vi "SubVI_1.vi"(9 "Step width":dbl=0.2, 10 "App":dbl=0.1, 11 "Points":i32=10) -> (3 "Disorder Pattern 2":dbl[](array[numeric]))   [LabVIEW 2019]
panel:
  in  "Set":bool
  in  "Generate":bool
  out "Disorder Pattern":dbl[](graph)=[1.0078411649904462, 1.0078411649904462, 0.9846991573254764, 0.9846991573254764, 0.9978814600222632, 0.9978814600222632, 0.9723089162683902, 0.9723089162683902, 1.011631648566163, 1.011631648566163]
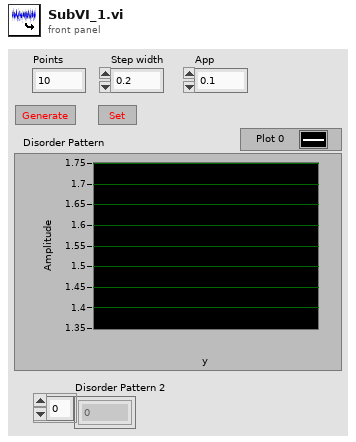
[diagram p1: front panel]
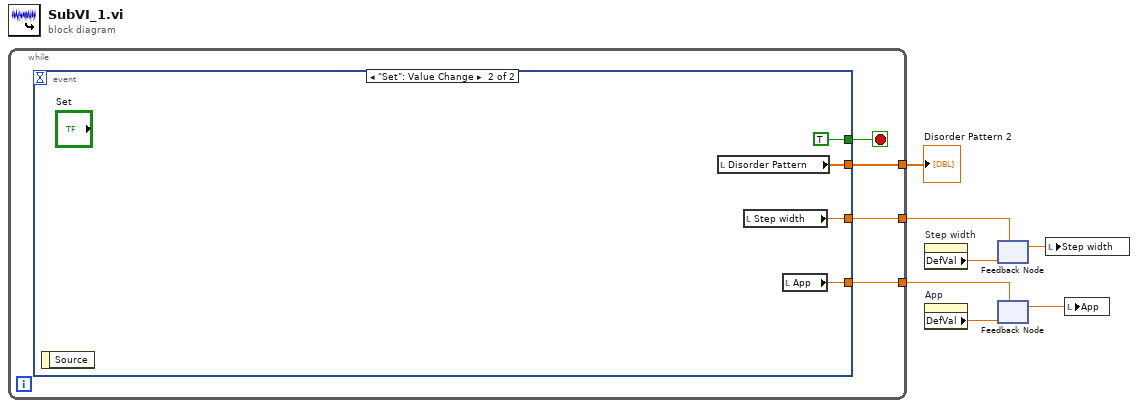
[diagram p0: block diagram]
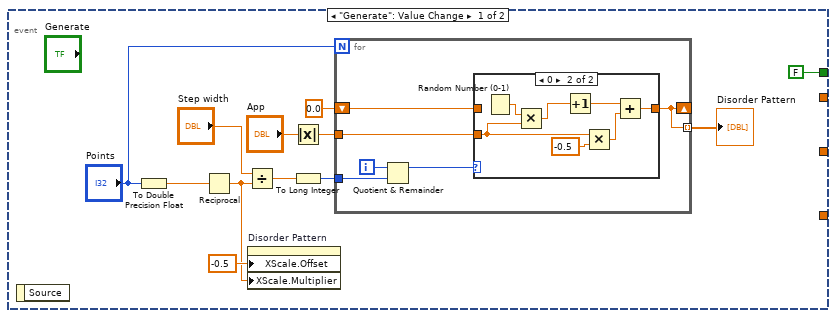
[diagram p2: hidden frame]
diagram:
  n1 = while {
    tunnel: [w10] -> w7
    tunnel: [w9] -> w4
    tunnel: [w8] -> w1
    stop <- w11 stop-if-true
    n2 = event shown="[1] \"Set\": Value Change" {
      selector: _ -> [_ _]
      dyn-events: _ -> [_ _]
      timeout: _ -> [_ _]
      tunnel: [FALSE TRUE] -> w11
      tunnel: [_ w41] -> w10
      tunnel: [_ w39] -> w9
      tunnel: [_ w38] -> w8
      event "Generate": Value Change {
        n3 = event-data() -> ()  [unwired: 1 in, 1 out]
        n4 = To Double Precision Float(number="Points") -> (double precision float=w17:dbl)
        n5 = Reciprocal(x=w17) -> (1/x=w12:dbl)
        n6 = Divide(x="Step width", y=w12) -> (x/y=w19:dbl)
        n7 = property on="Disorder Pattern" class="WFGraph (strict)"("XScale.Offset"=-0.5, "XScale.Multiplier"=w12) -> ()  [unwired: 2 in, 2 out]
        n8 = Absolute Value(x="App") -> (abs(x)=w23:dbl)
        n9 = To Long Integer(number=w19) -> (32bit integer=w21:i32)
        n10 = for {
          N: "Points" -> [_]
          tunnel: w21 -> [w28]
          tunnel: w23 -> [w27]
          shift-right: [w25] -> _
          shift-left: 0.0 -> [w26]
          tunnel: [w25] -> w15 mode=indexing
          i -> [w29]
          n11 = Quotient & Remainder(x=w29, y=w28) -> (x-y*floor(x/y)=w24:i32)  [unwired: 1 out]
          n12 = case shown="0" w24 {
            tunnel: w27 -> [_ w35]
            tunnel: [w30 w31] -> w25
            tunnel: w26 -> [w30 _]
            frame Default {
            }
            frame 0 {
              n13 = Random Number (0-1)() -> (number: 0 to 1=w37:dbl)
              n14 = Multiply(x=w37, y=w35) -> (x*y=w36:dbl)
              n15 = Increment(x=w36) -> (x+1=w33:dbl)
              n16 = Multiply(x=w35, y=-0.5) -> (x*y=w32:dbl)
              n17 = Add(x=w33, y=w32) -> (x+y=w31:dbl)
            }
          }
        }
        "Disorder Pattern" <- w15
      }
      event "Set": Value Change {
        n18 = event-data() -> ()  [unwired: 1 in, 1 out]
        n19 = local read "Disorder Pattern"() -> (w41:dbl[])
        n20 = local read "Step width"() -> (w39:dbl)
        n21 = local read "App"() -> (w38:dbl)
      }
    }
  }
  "Disorder Pattern 2" <- w7
  n22 = property on="Step width" class="DigNum (strict)"() -> ("DefVal"=w6:dbl)  [unwired: 2 in, 2 out]
  n23 = property on="App" class="DigNum (strict)"() -> ("DefVal"=w2:dbl)  [unwired: 2 in, 2 out]
  n24 = feedback-in #1(w4) -> ()
  n25 = feedback #1(w6) -> (w5:dbl)
  n26 = feedback #2(w2) -> (w3:dbl)
  n27 = feedback-in #2(w1) -> ()
  n28 = local write "Step width"(w5) -> ()
  n29 = local write "App"(w3) -> ()
